vi "Test ADC Rate (Direct).vi"() -> ()   [LabVIEW 2020, in "CTI-Scratchpad.lvlib"]
uses:
  CTI-Scratchpad.lvlib
  CTI/ADC Number.ctl
  CTI/VisaComms/VisaComms.lvclass
  <vilib>/ptbypt/NI_PtbyPt.lvlib
  CTI/CTI.lvlib
panel:
  in  "stop":bool
  out "ADC":dbl[][](graph)=[[2063.0, 0.0007534999895142391, 756.5504025676244]]
  in  "Port":refnum<visa-resource-name>="COM3"
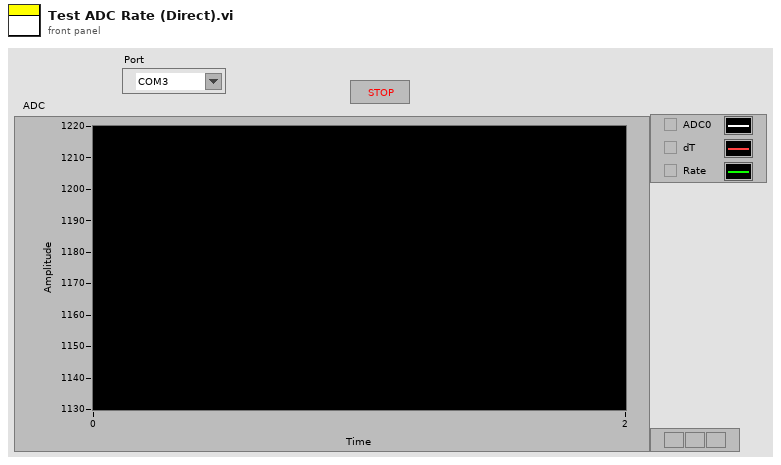
[diagram p1: front panel]
types:
  T1 = typedef "CTI.lvlib/ADC Number.ctl" = i8
  T2 = typedef "CTI.lvlib/Raw ADC.ctl" = u16
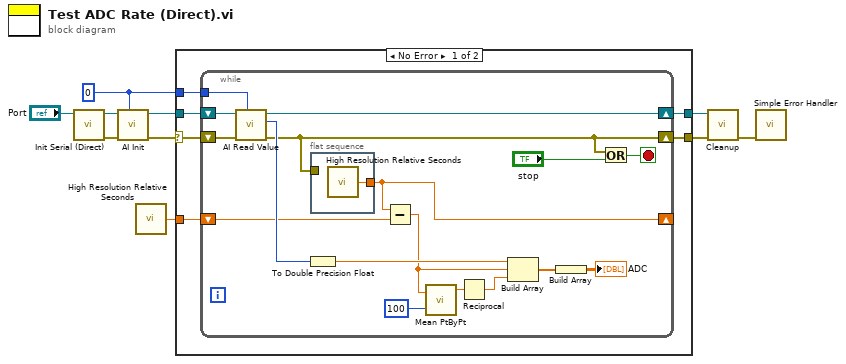
[diagram p0: block diagram]
diagram:
  w1 = T1 0 ("Channel")
  n1 = call "Init Serial (Direct).vi"("VISA resource name in"="Port") -> ("error out"=w8:errorcluster, "VisaComms out"=w9:refnum<class "VisaComms.lvclass">)  [unwired: 8 in, 1 out]
  n2 = call-dynamic "AI Init.vi"("ADC #"=w1, "error in (no error)"=w8, "VisaComms in"=w9) -> ("error out"=w7:errorcluster, "VisaComms out"=w2:refnum<class "VisaComms.lvclass">)  [unwired: 7 in]
  n3 = call <vilib>:"High Resolution Relative Seconds.vi"() -> ("relative seconds"=w3:dbl)
  n4 = case shown="No Error" w7 {
    selector: w7 -> [w14 w36]
    tunnel: w2 -> [w15 w35]
    tunnel: w1 -> [w16 _]
    tunnel: [w12 w36] -> w5
    tunnel: [w13 w35] -> w6
    tunnel: w3 -> [w11 _]
    frame No Error {
      n5 = while {
        tunnel: w16 -> [w17]
        shift-right: [w31] -> w13
        shift-left: w15 -> [w33]
        shift-right: [w27] -> w12
        shift-left: w14 -> [w32]
        shift-right: [w24] -> _
        shift-left: w11 -> [w25]
        stop <- w30 stop-if-true
        n6 = call-dynamic "AI Read Value.vi"("ADC #"=w17, "error in (no error)"=w32, "VisaComms in"=w33) -> ("error out"=w27:errorcluster, "Value"=w29:T2, "VisaComms out"=w31:refnum<class "VisaComms.lvclass">)  [unwired: 6 in]
        n7 = To Double Precision Float(number=w29) -> (double precision float=w23:dbl)
        n8 = flat-sequence {
          tunnel: w27 -> [_]
          tunnel: [w34] -> w24
          frame #0 {
            n9 = call <vilib>:"High Resolution Relative Seconds.vi"() -> ("relative seconds"=w34:dbl)
          }
        }
        n10 = Subtract(x=w24, y=w25) -> (x-y=w22:dbl)
        n11 = call <vilib>:"Mean PtByPt.vi"("x"=w22, "sample length"=100) -> ("mean"=w20:dbl)  [unwired: 2 in, 1 out]
        n12 = Reciprocal(x=w20) -> (1/x=w19:dbl)
        n13 = Build Array(w23, w22, w19) -> (w28:dbl[])
        n14 = Build Array(w28) -> (→"ADC":dbl[][])
        n15 = Or(x=w27, y="stop") -> (x .or. y?=w30:bool)
      }
    }
    frame Error {
    }
  }
  n16 = call-dynamic "Cleanup.vi"("error in (no error)"=w5, "VisaComms in"=w6) -> ("error out"=w4:errorcluster)  [unwired: 9 in]
  n17 = call <vilib>:"Simple Error Handler.vi"("error in (no error)"=w4) -> ()  [unwired: 4 in, 5 out]
